vi "AltZero.vi"(1 "z":dbl, 2 "x":dbl) -> (0 "y":dbl)   [LabVIEW 2012]
doc: "Squares a number and negates it according to input value."
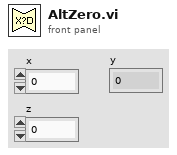
[diagram p1: front panel]
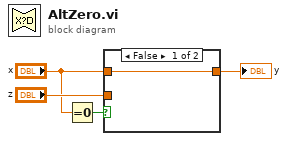
[diagram p0: block diagram]
diagram:
  n1 = Equal To 0?(x="x") -> (x = 0?=w2:bool)
  n2 = case shown="False" w2 {
    tunnel: [w5 w6] -> w4
    tunnel: "x" -> [w5 _]
    tunnel: "z" -> [_ w6]
    frame False {
    }
    frame True {
    }
  }
  "y" <- w4
